vi "JLT.vi"(0 "System no.":i32=1 min=1 max=4 step=1, 1 "Joystick ID":i32, 2 "Joystick axis":i32, 3 "Start point":i32=1, 4 "No.of digits":i16=4, 5 "error in":errorcluster, 6 "Factor":dbl[](array[numeric])) -> (14 "Controller error":bool, 19 "error out":errorcluster)   [LabVIEW 2020]
doc: "Sets joystick lookup table for a joystick connected to the controller. The amplitudes of the joystick axes are mapped to velocities of the controller axes. StartPoint is the start point in the lookup table, starting with 1. Valid values for Factor are -1.0 to 1.0 and define the factor which is applied to the currently set velocity (VEL in closed-loop operation, OVL in open-loop operation). No. of digits is the number of digits after the decimal point in the Factor value(s) that will be sent. Controller error is TRUE if selected system reports error code ? 0. Settings will not influence Joystick_Operation_Sample_Program.vi which works with a joystick connected to the host computer.\n\nE-709: Only supported if E-709 is used inside C-867K012/K013. Only one lookup table point for one axis per command allowed. To set more than one point you must create a for-loop around this VI. The joystick table consists of 256 points. The first point corresponds to the maximum joystick axis displacement in negative direction, the 256th point to the maximum displacement in positive direction.\n\nC-867, E-861, E-870, Mercury_GCS: Only one lookup table point for one joystick axis per command allowed. To set more than one point you must create a for-loop around this VI. The joystick table consists of 256 points. The first point corresponds to the maximum joystick axis displacement in negative direction, the 256th point to the maximum displacement in positive direction."
uses:
  whitespace.ctl
panel:
  # "Sets default lookup table for joysticks connected to the controller."
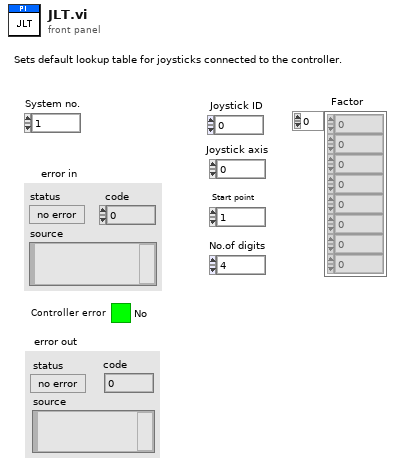
[diagram p1: front panel]
types:
  T1 = enum16{"Disable error check", "Force error check", "Use global settings"}
  T2 = typedef "whitespace.ctl" = u16
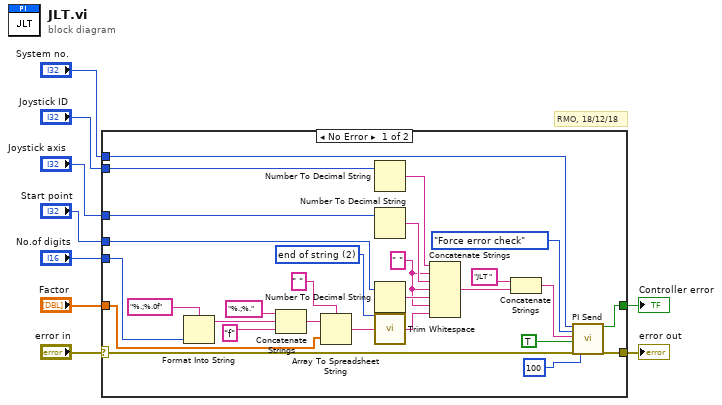
[diagram p0: block diagram]
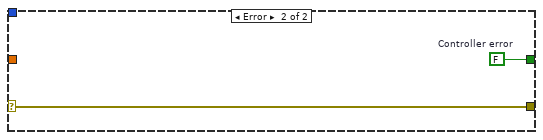
[diagram p2: hidden frame]
diagram:
  # "RMO, 18/12/18"
  n1 = case shown="No Error" "error in" {
    selector: "error in" -> [w14 w39]
    tunnel: [w10 w39] -> w9
    tunnel: "Factor" -> [w24 _]
    tunnel: "System no." -> [w37 _]
    tunnel: "Joystick ID" -> [w36 _]
    tunnel: "Joystick axis" -> [w32 _]
    tunnel: "Start point" -> [w31 _]
    tunnel: "No.of digits" -> [w28 _]
    tunnel: [w11 w38] -> w1
    frame No Error {
      w22 = T2 2 items=["both", "start of string", "end of string"] ("location (both)")
      w17 = " " ("string")
      n2 = Format Into String(format string="%.;%.0f" ("Format String"), w28) -> (resulting string=w27:string)  [unwired: 2 in, 1 out]
      n3 = Concatenate Strings("%.;%." ("Format String"), w27, "f" ("Format String")) -> (w25:string)
      n4 = Array To Spreadsheet String(delimiter (Tab)=" ", array=w24, 3:w25) -> (spreadsheet string=w21:string)
      n5 = Number To Decimal String(number=w36) -> (decimal integer string=w20:string)  [unwired: 1 out]
      n6 = Number To Decimal String(number=w32) -> (decimal integer string=w19:string)  [unwired: 1 out]
      n7 = Number To Decimal String(number=w31) -> (decimal integer string=w18:string)  [unwired: 1 out]
      n8 = call "Trim Whitespace.vi"("string"=w21, "location (both)"=w22) -> ("trimmed string"=w16:string)
      n9 = Concatenate Strings(w20, w17, w19, w17, w18, w17, w16) -> (w15:string)
      n10 = Concatenate Strings("JLT ", w15) -> (w33:string)
      n11 = call "PI Send.vi"("System no."=w37, "Error check settings"=T1."Force error check", "String to send"=w33, "Attach termination char.?"=TRUE ("Attach Linefeed?"), "error in"=w14, "Delay before error check (ms)"=u32 100 ("milliseconds to wait")) -> ("Controller error"=w11:bool, "error out"=w10:errorcluster)  [unwired: 12 out]
    }
    frame Error {
      w38 = FALSE  # Controller error
    }
  }
  "error out" <- w9
  "Controller error" <- w1
